vi "cam_get image.vi"(8 "error in (no error)":errorcluster, 9 "camera image":T4, 10 "camera ref":refnum<k20>, 11 "SceneGraphDisplay in":refnum<vi>) -> (0 "error out":errorcluster, 1 "height":sgl, 3 "Refnum out":T4, 4 "Rectangle.right":i16, 6 "Rectangle.bottom":i16)   [LabVIEW 2018]
uses:
  <vilib>/vision/Image Controls.llb/IMAQ Image.ctl
  <resource>/objmgr/LVODE.rc
panel:
  out "cluster 3":T1
  out "cluster 2":T2
  out "cluster":T3
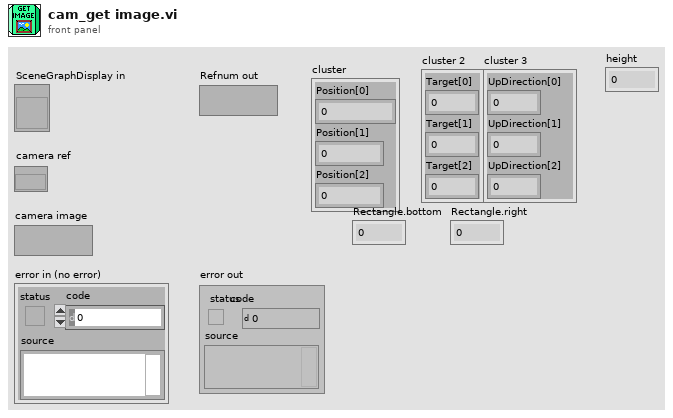
[diagram p1: front panel]
types:
  T1 = cluster{"UpDirection[0]":sgl, "UpDirection[1]":sgl, "UpDirection[2]":sgl}
  T2 = cluster{"Target[0]":sgl, "Target[1]":sgl, "Target[2]":sgl}
  T3 = cluster{"Position[0]":sgl, "Position[1]":sgl, "Position[2]":sgl}
  T4 = typedef "IMAQ Image.ctl" = refnum<image>
  T5 = typedef "imagedata.ctl" = cluster{"image type":i32, "image depth":i32, "image":u8[], "mask":u8[], "colors":u32[], "Rectangle":cluster{"left":i16, "top":i16, "right":i16, "bottom":i16}}
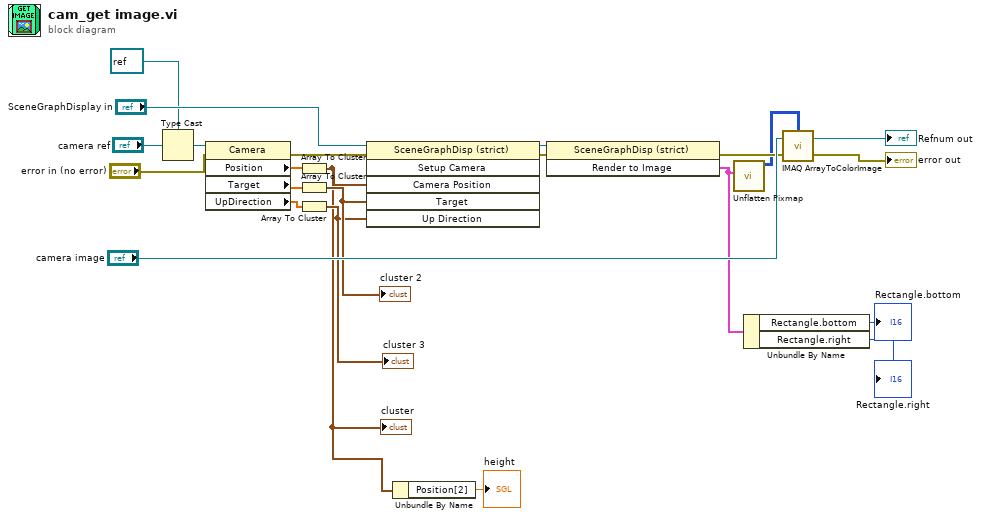
[diagram p0: block diagram]
diagram:
  n1 = Type Cast(type=refnum<k20> refnum ("Camera"), x="camera ref") -> (*(type *) &x=w11:refnum<k20>)
  n2 = property class="Camera"(reference=w11, error in="error in (no error)") -> (error out=w14:errorcluster, "Position"=w8:sgl[], "Target"=w9:sgl[], "UpDirection"=w10:sgl[])  [unwired: 1 out]
  n3 = Array To Cluster(array=w8) -> (cluster=w2:T3)
  "cluster" <- w2
  n4 = Array To Cluster(array=w9) -> (cluster=w7:T2)
  "cluster 2" <- w7
  n5 = Array To Cluster(array=w10) -> (cluster=w6:T1)
  "cluster 3" <- w6
  n6 = invoke class="SceneGraphDisp (strict)" method="Setup Camera"(reference="SceneGraphDisplay in", error in=w14, "Camera Position"=w2, "Target"=w7, "Up Direction"=w6) -> (reference out=w16:refnum<vi>, error out=w17:errorcluster)  [unwired: 1 in, 4 out]
  n7 = Unbundle By Name(w2) -> ("Position[2]"=→"height":sgl)
  n8 = invoke class="SceneGraphDisp (strict)" method="Render to Image"(reference=w16, error in=w17) -> (error out=w18:errorcluster, "Get Image"=w5:T5)  [unwired: 1 in, 1 out]
  n9 = call <vilib>:"Unflatten Pixmap.vi"("image data"=w5) -> ("24-bit pixmap"=w15:u32[][])  [unwired: 4 in, 6 out]
  n10 = Unbundle By Name(w5) -> ("Rectangle.bottom"=→"Rectangle.bottom":i16, "Rectangle.right"=→"Rectangle.right":i16)
  n11 = call "IMAQ ArrayToColorImage"("Image Pixels (U32)"=w15, "Image"="camera image", "error in (no error)"=w18) -> ("Image Out"=→"Refnum out":T4, "error out"=→"error out":errorcluster)  [unwired: 2 in]
